vi "Read CSV File.vi"(8 "error in (no error)":errorcluster, 11 "Path":path) -> (0 "error out":errorcluster, 3 "Data":dbl[](array[numeric]))   [LabVIEW 2020]
uses:
  <vilib>/Utility/file.llb/Read Delimited Spreadsheet (DBL).vi
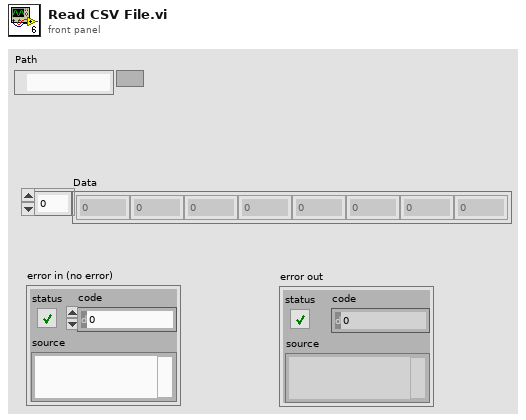
[diagram p1: front panel]
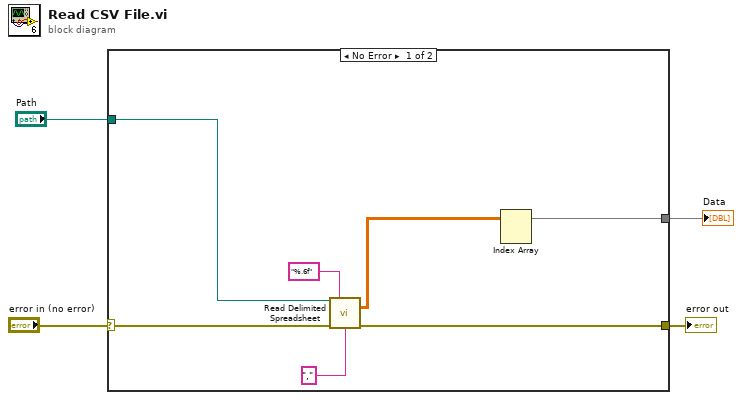
[diagram p0: block diagram]
diagram:
  n1 = case shown="No Error" "error in (no error)" {
    selector: "error in (no error)" -> [w8 w12]
    tunnel: "Path" -> [w9 _]
    tunnel: [w7 w12] -> w2
    tunnel: [w5 _] -> w1
    frame No Error {
      n2 = call-poly <vilib>:"Read Delimited Spreadsheet.vi"("file path (dialog if empty)"=w9, "format (%.3f)"="%.6f", "error in (no error)"=w8, "delimiter (\\t)"="," ("delimiter (\\t)")) -> ("all rows"=w6:dbl[][], "error out"=w7:errorcluster)  [unwired: 6 in, 4 out]
      n3 = Index Array(array=w6) -> (element=w5:dbl[])  [unwired: 2 in]
    }
    frame Error {
    }
  }
  "error out" <- w2
  "Data" <- w1
